vi "move.vi"(8 "error in (no error)":errorcluster, 11 "DL090409StageScaffold in":refnum<class "StageMMS2015ASIfromScientifica.lvclass">) -> (0 "error out":errorcluster, 3 "DL090409StageScaffold out":refnum<class "StageMMS2015ASIfromScientifica.lvclass">)   [LabVIEW 2010, in "StageMMS2015ASIfromScientifica.lvclass"]
uses:
  StageMMS2015ASIfromScientifica.lvclass
  StageDL090409Scaffold/StageDL090409Scaffold/StageDL090409Scaffold.lvclass
  common/classes/ErrorController/ErrorController/class_data.vi
  common/classes/ErrorController/ErrorController/ErrorController.lvclass
  common/classes/SpaceVector/SpaceVector/SpaceVector.lvclass
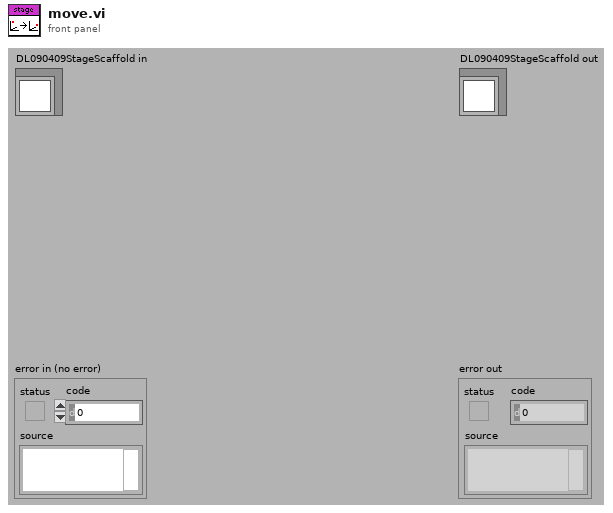
[diagram p1: front panel]
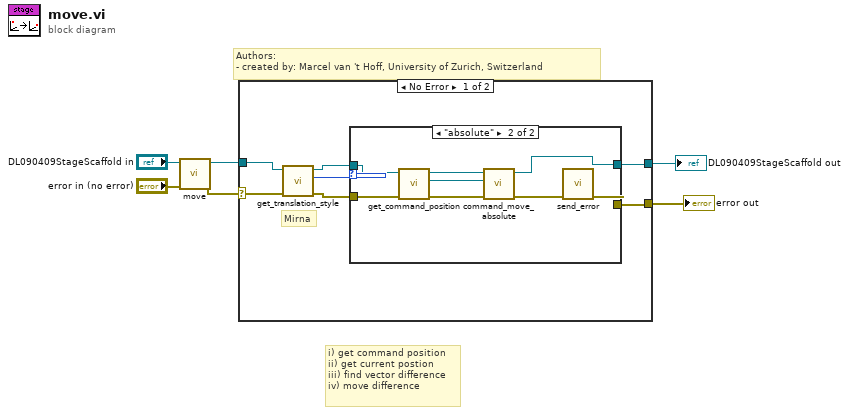
[diagram p0: block diagram]
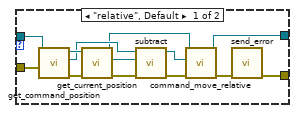
[diagram p2: hidden frame]
diagram:
  # "i) get command position\nii) get current postion\niii) find vector difference\niv) move difference"
  # "Authors: \n- created by: Marcel van 't Hoff, University of Zurich, Switzerland"
  n1 = call-parent "move.vi"("error in (no error)"="error in (no error)", "DL090409StageScaffold in"="DL090409StageScaffold in") -> ("error out"=w4:errorcluster, "DL090409StageScaffold out"=w3:refnum<class "StageMMS2015ASIfromScientifica.lvclass">)  [unwired: 8 in]
  n2 = case shown="No Error" w4 {
    selector: w4 -> [w8 w36]
    tunnel: [w13 w36] -> w2
    tunnel: [w12 w35] -> w1
    tunnel: w3 -> [w11 w35]
    frame No Error {
      # "Mirna"
      n3 = call-dynamic "get_translation_style.vi"("error in (no error)"=w8, "StageDL090409Scaffold in"=w11) -> ("error out"=w9:errorcluster, "translation style"=w7:enum16{"relative", "absolute"}, "StageDL090409Scaffold out"=w10:refnum<class "StageMMS2015ASIfromScientifica.lvclass">)  [unwired: 7 in]
      n4 = case shown="\"absolute\"" w7 {
        tunnel: [w26 w32] -> w13
        tunnel: [w25 w31] -> w12
        tunnel: w10 -> [w15 w34]
        tunnel: w9 -> [w14 w33]
        frame "relative", Default {
          n5 = call-dynamic "get_command_position.vi"("error in (no error)"=w14, "DL090409StageScaffold.lvclass in"=w15) -> ("error out"=w24:errorcluster, "SpaceVector.lvclass"=w22:refnum<class "SpaceVector.lvclass">, "DL090409StageScaffold.lvclass out"=w23:refnum<class "StageMMS2015ASIfromScientifica.lvclass">)  [unwired: 7 out]
          n6 = call-dynamic "get_current_position.vi"("error in (no error)"=w24, "DL090409StageScaffold.lvclass in"=w23) -> ("error out"=w20:errorcluster, "current position"=w21:refnum<class "SpaceVector.lvclass">, "DL090409StageScaffold.lvclass out"=w17:refnum<class "StageMMS2015ASIfromScientifica.lvclass">)  [unwired: 7 in]
          n7 = call "subtract.vi"("error in (no error)"=w20, "subtrahend"=w21, "SpaceVector in"=w22) -> ("error out"=w18:errorcluster, "SpaceVector out"=w19:refnum<class "SpaceVector.lvclass">)  [unwired: 7 in]
          n8 = call-dynamic "command_move_relative.vi"("error in (no error)"=w18, "target  position"=w19, "StageMH110930Scientifica in"=w17) -> ("error out"=w16:errorcluster, "StageMH110930Scientifica out"=w25:refnum<class "StageMMS2015ASIfromScientifica.lvclass">)  [unwired: 7 in]
          n9 = call "send_error.vi"("error in (no error)"=w16) -> ("error out"=w26:errorcluster)  [unwired: 10 in]
        }
        frame "absolute" {
          n10 = call-dynamic "get_command_position.vi"("error in (no error)"=w33, "DL090409StageScaffold.lvclass in"=w34) -> ("error out"=w28:errorcluster, "SpaceVector.lvclass"=w29:refnum<class "SpaceVector.lvclass">, "DL090409StageScaffold.lvclass out"=w30:refnum<class "StageMMS2015ASIfromScientifica.lvclass">)  [unwired: 7 out]
          n11 = call-dynamic "command_move_absolute.vi"("error in (no error)"=w28, "target  position"=w29, "StageMH110930Scientifica in"=w30) -> ("error out"=w27:errorcluster, "StageMH110930Scientifica out"=w31:refnum<class "StageMMS2015ASIfromScientifica.lvclass">)  [unwired: 7 in]
          n12 = call "send_error.vi"("error in (no error)"=w27) -> ("error out"=w32:errorcluster)  [unwired: 10 in]
        }
      }
    }
    frame Error {
    }
  }
  "error out" <- w2
  "DL090409StageScaffold out" <- w1
